vi "round to one sig fig.vi"(1 "input number":dbl) -> (0 "rounded to 1 sig fig":dbl)   [LabVIEW 2023]
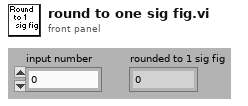
[diagram p1: front panel]
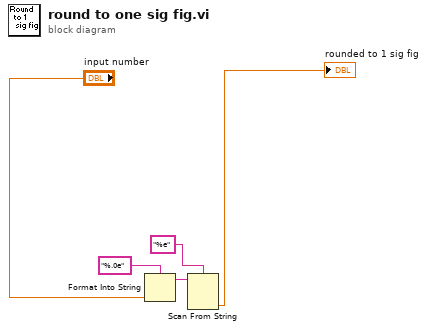
[diagram p0: block diagram]
diagram:
  n1 = Format Into String(format string="%.0e", "input number") -> (resulting string=w3:string)  [unwired: 2 in, 1 out]
  n2 = Scan From String(format string="%e", input string=w3) -> (output 1=→"rounded to 1 sig fig":dbl)  [unwired: 2 in, 4 out]
